vi "parse_colors.vi"(11 "Numeric":i32) -> (3 "Cluster":cluster{"Red":i32, "Green":i32, "Blue":i32})   [LabVIEW 2014]
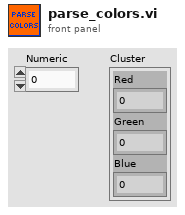
[diagram p1: front panel]
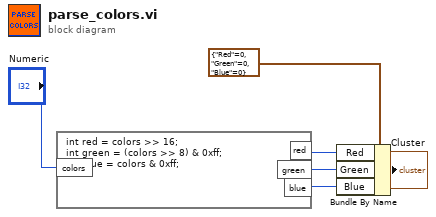
[diagram p0: block diagram]
diagram:
  n1 = formula code="int red = colors >> 16;\nint green = (colors >> 8) & 0xff;\nint blue = colors & 0xff;"("colors"="Numeric") -> ("red"=w2:i32, "green"=w6:i32, "blue"=w3:i32)
  n2 = Bundle By Name(cluster=cluster{"Red":i32, "Green":i32, "Blue":i32} {"Red"=0, "Green"=0, "Blue"=0}, "Red"=w2, "Green"=w6, "Blue"=w3) -> (→"Cluster":cluster{"Red":i32, "Green":i32, "Blue":i32})
